vi "PerisPump_set speed.vi"(1 "Speed (rpm)":string="20") -> ()   [LabVIEW 2023]
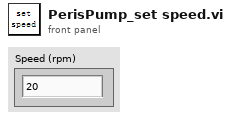
[diagram p1: front panel]
types:
  T1 = enum16{"Query address", "Set address", "Set speed", "Clockwise rotation", "Counterclockwise rotation", "Stop"}
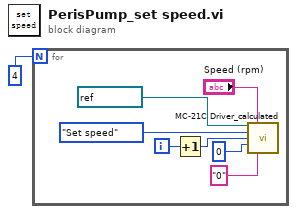
[diagram p0: block diagram]
diagram:
  n1 = for {
    N: 4 -> [_]
    i -> [w4]
    n2 = Increment(x=w4) -> (x+1=w3:i32)
    n3 = call "MC-21C Driver_calculated.vi"("Peristaltic Pump COM"=refnum<visa-resource-name> "COM3", "Speed (rpm)"="Speed (rpm)", "Operation"=T1."Set speed", "Address"=w3, "Set address (0-255)"=i16 0, "Step"="0") -> ()  [unwired: 7 in, 3 out]
  }
